vi "setpoint and rotate.vi"(0 "axis 1: sp position °":dbl, 1 "m/c temp setpoint":dbl, 5 "move axis 1":bool, 7 "axis 2: sp position °":dbl, 9 "move axis 2":bool, 11 "error in":errorcluster) -> (4 "Status OUT":T1, 15 "error out":errorcluster)   [LabVIEW 2016]
panel:
  out "m/c temp":dbl
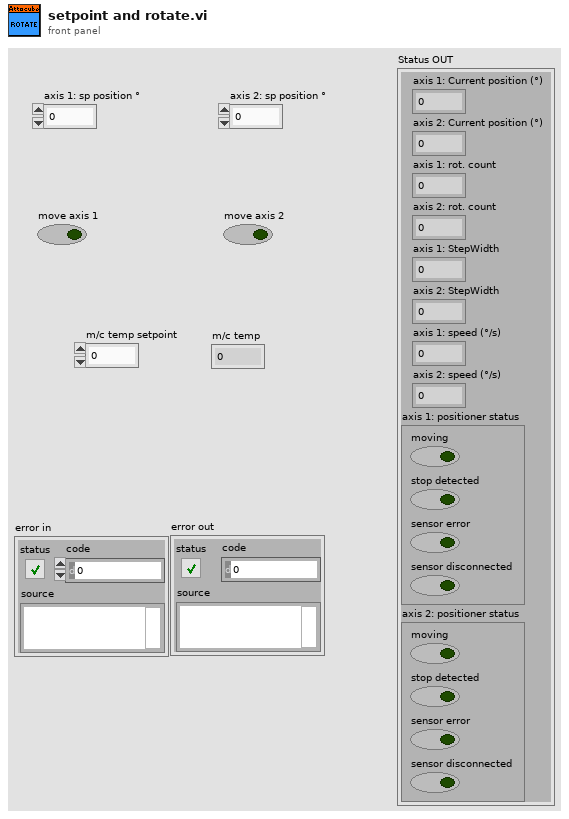
[diagram p1: front panel]
types:
  T1 = cluster{"axis 1: Current position (°)":dbl, "axis 2: Current position (°)":dbl, "axis 1: rot. count":dbl, "axis 2: rot. count":dbl, "axis 1: StepWidth":dbl, "axis 2: StepWidth":dbl, "axis 1: speed (°/s)":dbl, "axis 2: speed (°/s)":dbl, "axis 1: positioner status":cluster{"moving":bool, "stop detected":bool, "sensor error":bool, "sensor disconnected":bool}, "axis 2: positioner status":cluster{"moving":bool, "stop detected":bool, "sensor error":bool, "sensor disconnected":bool}}
  T2 = cluster{"axis 1: Absolute":bool, "axis 2: Absolute":bool, "axis 1: Stop moving":bool, "axis 2: Stop moving":bool, "axis 1: Output":bool, "axis 2: Output":bool, "set static amplitude\nwhen moving":bool}
  T3 = cluster{"axis 1: Amplitude [V]":dbl, "axis 2: Amplitude [V]":dbl, "axis 1: DCLevel [V]":dbl, "axis 2: DCLevel [V]":dbl, "axis 1: Frequency [Hz]":dbl, "axis 2: Frequency [Hz]":dbl, "axis 1: sp position °":dbl, "axis 2: sp position °":dbl, "axis 1: sp rot count":dbl, "axis 2: sp rot count":dbl}
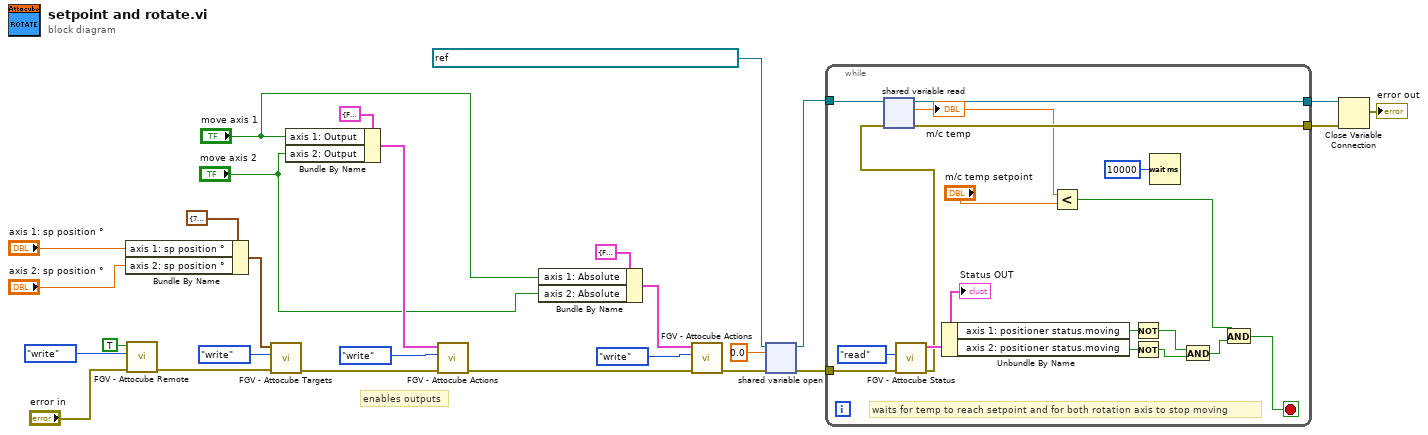
[diagram p0: block diagram]
diagram:
  # "enables outputs"
  n1 = Bundle By Name(cluster=T3 {"axis 1: Amplitude [V]"=70.0, "axis 2: Amplitude [V]"=0.0, "axis 1: DCLevel [V]"=0.0, "axis 2: DCLevel [V]"=0.0, "axis 1: Frequency [Hz]"=3500.0, "axis 2: Frequency [Hz]"=3500.0, "axis 1: sp position °"=230.0, "axis 2: sp position °"=255.0, "axis 1: sp rot count"=0.0, "axis 2: sp rot count"=0.0} ("Targets In"), "axis 1: sp position °"="axis 1: sp position °", "axis 2: sp position °"="axis 2: sp position °") -> (w22:T3)
  n2 = call "FGV - Attocube Remote.vi"("error in"="error in", "Function"=enum16{"write", "read"}."write", "Attocube Remote"=TRUE) -> ("error out"=w25:errorcluster)  [unwired: 3 in, 1 out]
  n3 = call "FGV - Attocube Targets.vi"("error in"=w25, "Function"=enum16{"write", "read"}."write", "Targets In"=w22) -> ("error out"=w12:errorcluster)  [unwired: 3 in, 1 out]
  n4 = Bundle By Name(cluster=T2 {"axis 1: Absolute"=FALSE, "axis 2: Absolute"=FALSE, "axis 1: Stop moving"=FALSE, "axis 2: Stop moving"=FALSE, "axis 1: Output"=FALSE, "axis 2: Output"=FALSE, "set static amplitude\nwhen moving"=FALSE} ("Actions IN"), "axis 1: Output"="move axis 1", "axis 2: Output"="move axis 2") -> (w17:T2)
  n5 = call "FGV - Attocube Actions.vi"("error in"=w12, "Function"=enum16{"write", "read"}."write", "Actions IN"=w17) -> ("error out"=w11:errorcluster)  [unwired: 3 in, 1 out]
  n6 = Bundle By Name(cluster=T2 {"axis 1: Absolute"=FALSE, "axis 2: Absolute"=FALSE, "axis 1: Stop moving"=FALSE, "axis 2: Stop moving"=FALSE, "axis 1: Output"=FALSE, "axis 2: Output"=FALSE, "set static amplitude\nwhen moving"=FALSE} ("Actions IN"), "axis 1: Absolute"="move axis 1", "axis 2: Absolute"="move axis 2") -> (w14:T2)
  n7 = call "FGV - Attocube Actions.vi"("error in"=w11, "Function"=enum16{"write", "read"}."write", "Actions IN"=w14) -> ("error out"=w8:errorcluster)  [unwired: 3 in, 1 out]
  n8 = shared-variable-open(refnum<k21> "ni.var.psp://housesoftheholy/MNK_18T/MNK_TC_T3" ("shared variable refnum in"), w8, 0.0) -> (w6:refnum<k21>, w7:errorcluster)  [unwired: 1 in]
  n9 = while {
    tunnel: w7 -> [w42]
    tunnel: w6 -> [w36]
    tunnel: [w35] -> w5
    tunnel: [w34] -> w4
    stop <- w29 stop-if-true
    # "waits for temp to reach setpoint and for both rotation axis to stop moving"
    n10 = call "FGV - Attocube Status.vi"("error in"=w42, "Function"=enum16{"write", "read"}."read") -> ("error out"=w37:errorcluster, "Status OUT"=w44:T1)  [unwired: 4 in]
    "Status OUT" <- w44
    n11 = shared-variable-read(w36, w37) -> (w35:refnum<k21>, w34:errorcluster, w33:dbl)  [unwired: 1 out]
    "m/c temp" <- w33
    n12 = Unbundle By Name(w44) -> ("axis 1: positioner status.moving"=w41:bool, "axis 2: positioner status.moving"=w40:bool)
    n13 = Less?(x=w33, y="m/c temp setpoint") -> (x < y?=w31:bool)
    n14 = Not(x=w41) -> (.not. x?=w39:bool)
    n15 = Not(x=w40) -> (.not. x?=w38:bool)
    n16 = Wait (ms)(milliseconds to wait=u32 10000) -> ()  [unwired: 1 out]
    n17 = And(x=w39, y=w38) -> (x .and. y?=w30:bool)
    n18 = And(x=w31, y=w30) -> (x .and. y?=w29:bool)
  }
  n19 = Close Variable Connection(8:w4, 11:w5) -> (0:→"error out":errorcluster)
